vi "set_output_mode.vi"(8 "error in (no error)":errorcluster, 10 "Ouptut mode":T1="0", 11 "connection ID":refnum<k5>) -> (0 "error out":errorcluster, 3 "connection ID out":refnum<k5>)   [LabVIEW 2018]
uses:
  typedefs/output_mode.ctl
panel:
  out "bytes written":i32
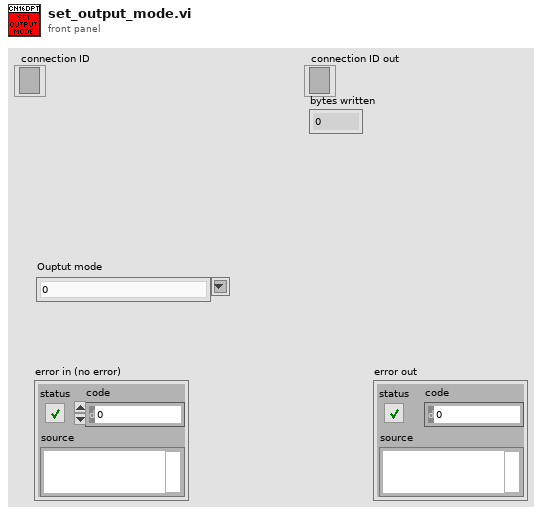
[diagram p1: front panel]
types:
  T1 = typedef "output_mode.ctl" = string
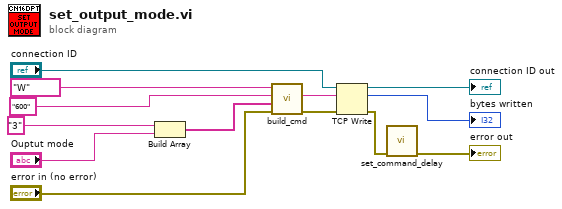
[diagram p0: block diagram]
diagram:
  n1 = Build Array("3" ("element"), "Ouptut mode") -> (w7:T1[])
  n2 = call "build_cmd.vi"("error in (no error)"="error in (no error)", "Parameter list"=w7, "Command ID"="600", "Command class"="W") -> ("error out"=w10:errorcluster, "Command"=w9:string)  [unwired: 6 in]
  n3 = TCP Write(connection ID="connection ID", data in=w9, error in (no error)=w10) -> (connection ID out=→"connection ID out":refnum<k5>, bytes written=→"bytes written":i32, error out=w2:errorcluster)  [unwired: 1 in]
  n4 = call "set_command_delay.vi"("error in (no error)"=w2) -> ("error out"=→"error out":errorcluster)  [unwired: 10 in]
